vi "Searching connected instruments.vi"(8 "error in (no error)":errorcluster) -> (0 "error out":errorcluster, 2 "Found Instruments":string[][](array[string]))   [LabVIEW 2020, in "Test Framework.lvclass"]
doc: "Finds all connected instruments and gets its IDN.\nFor comport it verifies that a PIC board is connected."
uses:
  Test Framework.lvclass
  <vilib>/Instr/_visa.llb/VISA Find Search Mode.ctl
  <vilib>/Instr/_visa.llb/VISA Configure Serial Port (Instr).vi
panel:
  out "read buffer 2":string
  in  "Cancel":bool
  out "read buffer":string
  out "Searching Instruments":u8(slide) scale=0.0..100.0
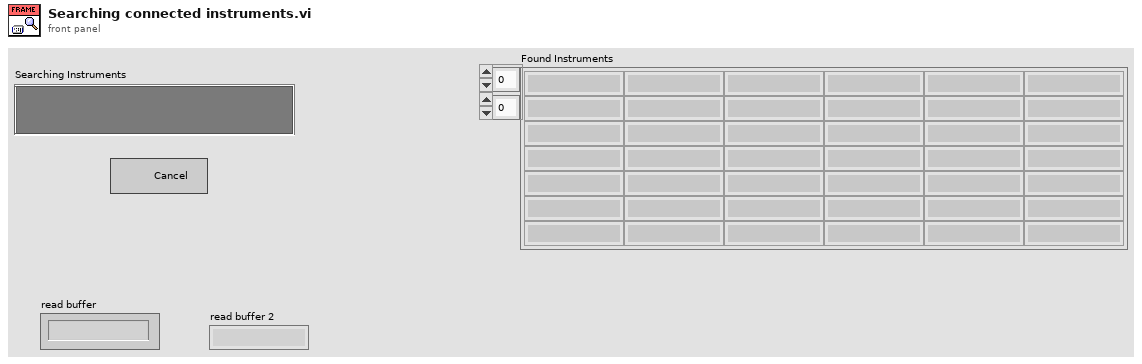
[diagram p1: front panel]
types:
  T1 = typedef "VISA Find Search Mode.ctl" = u32
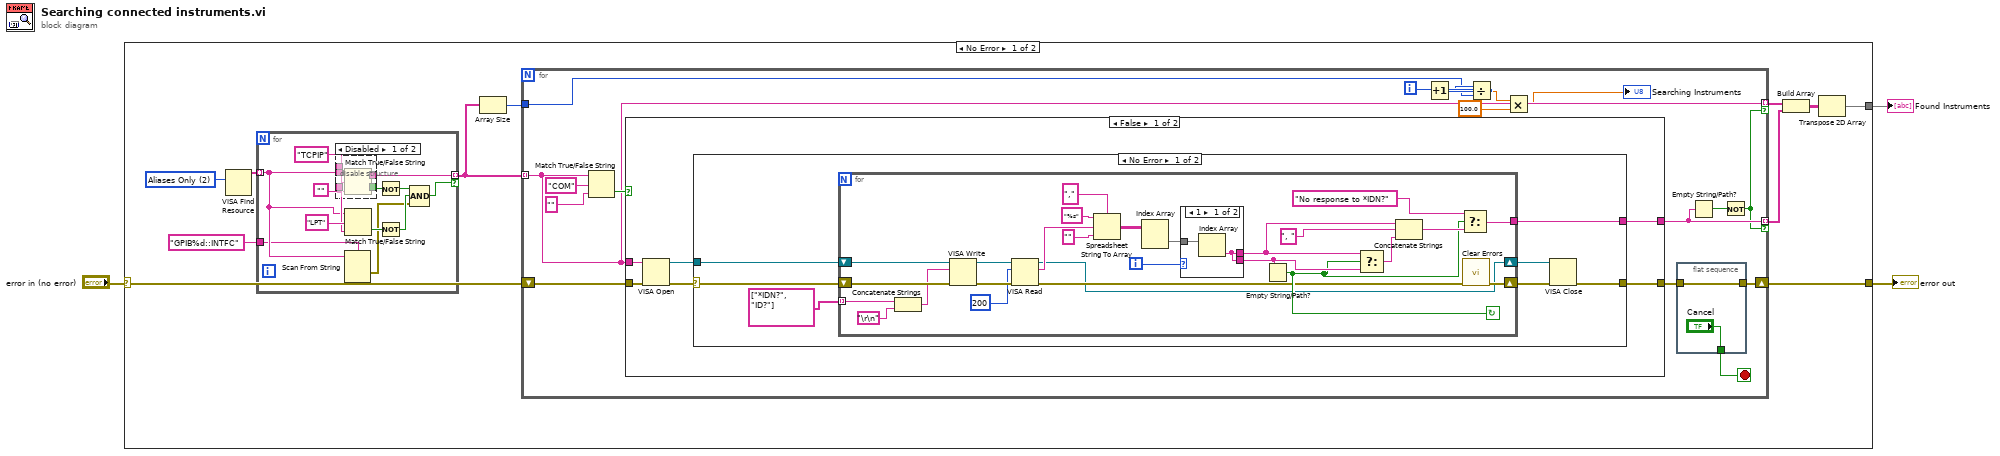
[diagram p0: block diagram]
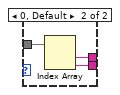
[diagram p2: hidden frame]
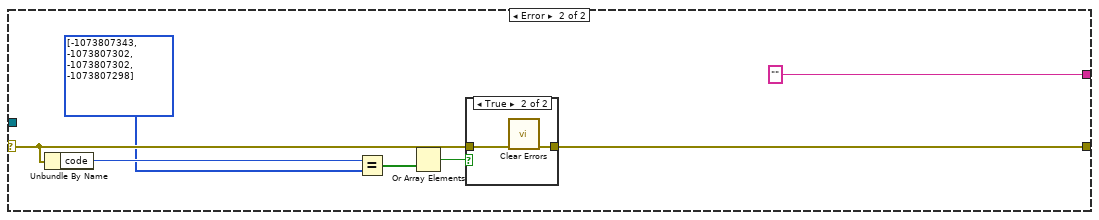
[diagram p3: hidden frame]
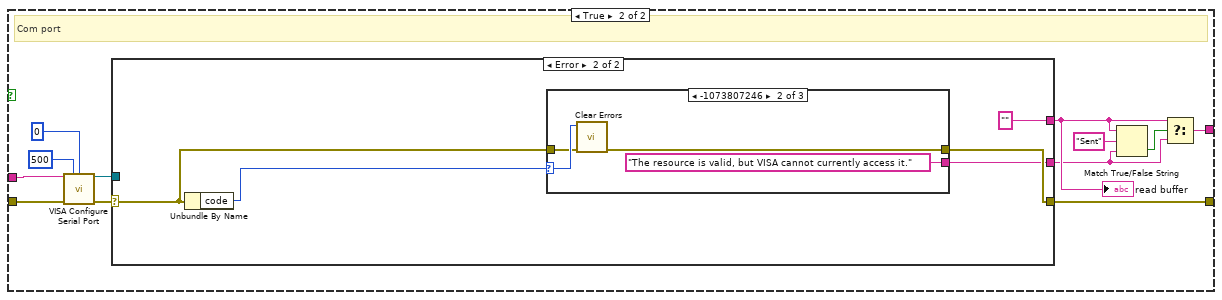
[diagram p5: hidden frame]
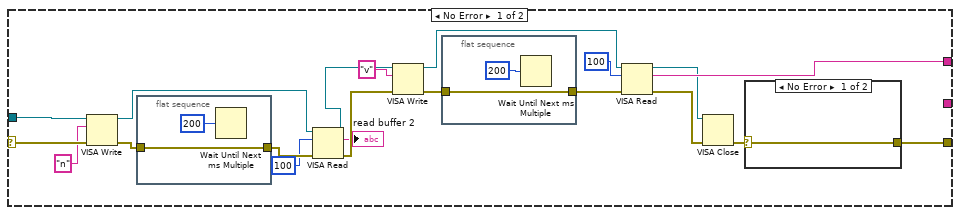
[diagram p6: hidden frame]
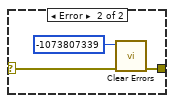
[diagram p7: hidden frame]
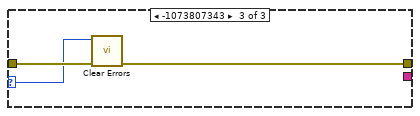
[diagram p9: hidden frame]
diagram:
  n1 = case shown="No Error" "error in (no error)" {
    selector: "error in (no error)" -> [w8 w159]
    tunnel: [w7 w159] -> w2
    tunnel: [w9 _] -> w1
    frame No Error {
      w14 = T1 2 items=["Canonical Names Only"=0, "Aliases Only"=2, "Include Matching Aliases"=3, "Include All Aliases"=4] ("Search Mode")
      n2 = VISA Find Resource(10:w14) -> (3:w13:string[])  [unwired: 2 in, 2 out]
      n3 = for {
        tunnel: w13 -> [w142] mode=indexing
        tunnel: [w152] -> w6 mode=indexing if=w145
        tunnel: "GPIB%d::INTFC" ("true string") -> [w141]
        w144 = ""
        n4 = disable-structure shown="Disabled" {
          disable-tunnel: [w157 w158] -> w152
          disable-tunnel: [w156 _] -> w151
          disable-tunnel: "TCPIP" ("true string") -> [w155 _]
          disable-tunnel: w144 -> [w154 _]
          disable-tunnel: w142 -> [w153 w158]
          frame Disabled {
            n5 = Match True/False String(2:w154, 3:w155, 4:w153) -> (0:w156:bool, 1:w157:string)
          }
          frame Enabled {
          }
        }
        n6 = Scan From String(format string=w141, input string=w142) -> (error out=w143:errorcluster)  [unwired: 4 in, 2 out]
        n7 = Match True/False String(2:w144, 3:"LPT" ("true string"), 4:w142) -> (0:w148:bool)  [unwired: 1 out]
        n8 = Not(x=w151) -> (.not. x?=w147:bool)
        n9 = Not(x=w148) -> (.not. x?=w146:bool)
        n10 = Compound Arithmetic op=AND(w147, w146, w143) -> (w145:bool)
      }
      n11 = Array Size(array=w6) -> (size(s)=w5:i32)
      n12 = for {
        tunnel: w6 -> [w27] mode=indexing
        tunnel: [w26] -> w11 mode=indexing if=w25
        shift-right: [w16] -> w7
        shift-left: w8 -> [w28]
        tunnel: [w27] -> w12 mode=indexing if=w25
        tunnel: w5 -> [w21]
        i -> [w23]
        stop <- w17 stop-if-true
        n13 = Match True/False String(2:"" ("false string"), 3:"COM" ("true string"), 4:w27) -> (0:w29:bool)  [unwired: 1 out]
        n14 = case shown="False" w29 {
          tunnel: w27 -> [w39 w99]
          tunnel: [w37 w91] -> w26
          tunnel: [w35 w94] -> w15
          tunnel: w28 -> [w34 w95]
          frame False {
            n15 = VISA Open(error in (no error)=w34, VISA resource name=w39) -> (VISA resource name=w38:refnum<visa-resource-name>, error out=w36:errorcluster)  [unwired: 3 in]
            n16 = case shown="No Error" w36 {
              selector: w36 -> [w45 w82]
              tunnel: w38 -> [w46 _]
              tunnel: [w44 ""] -> w37
              tunnel: [w41 w81] -> w35
              frame No Error {
                n17 = for {
                  tunnel: [w57] -> w44
                  shift-right: [w59] -> w42
                  shift-left: w45 -> [w62]
                  tunnel: string[] ["*IDN?", "ID?"] -> [w55] mode=indexing
                  shift-right: [w47] -> w40
                  shift-left: w46 -> [w69]
                  i -> [w49]
                  stop <- w50 continue-if-true
                  n18 = Concatenate Strings(w55, "\r\n") -> (w61:string)
                  n19 = VISA Write(VISA resource name=w69, write buffer=w61, error in (no error)=w62) -> (VISA resource name out=w71:refnum<visa-resource-name>, error out=w72:errorcluster)  [unwired: 1 out]
                  n20 = VISA Read(VISA resource name=w71, byte count=u32 200, error in (no error)=w72) -> (VISA resource name out=w47:refnum<visa-resource-name>, read buffer=w51:string, error out=w48:errorcluster)  [unwired: 1 out]
                  n21 = Spreadsheet String To Array(delimiter (Tab)=",", format string="%s", spreadsheet string=w51, array type (2D Dbl)="") -> (array=w66:string[][])
                  n22 = Index Array(array=w66) -> (element=w65:string[])  [unwired: 2 in]
                  n23 = case shown="1" w49 {
                    tunnel: w65 -> [w74 w77]
                    tunnel: [w73 w76] -> w54
                    tunnel: [w73 w75] -> w53
                    frame 1 {
                      n24 = Index Array(array=w74) -> (element=w73:string)  [unwired: 1 in]
                    }
                    frame 0, Default {
                      n25 = Index Array(array=w77) -> (element #1=w76:string, element #2=w75:string)  [unwired: 2 in]
                    }
                  }
                  n26 = Empty String/Path?(string/path=w53) -> (empty?=w50:bool)
                  n27 = Select(t=w54, s=w50, f=w53) -> (s? t:f=w52:string)
                  n28 = Concatenate Strings(w54, ", ", w52) -> (w58:string)
                  n29 = Select(t="No response to *IDN?", s=w50, f=w58) -> (s? t:f=w57:string)
                  n30 = call <vilib>:"Clear Errors.vi"("error in (no error)"=w48) -> ("error out"=w59:errorcluster)  [unwired: 5 in, 1 out]
                }
                n31 = VISA Close(VISA resource name=w40, error in (no error)=w42) -> (error out=w41:errorcluster)
              }
              frame Error {
                n32 = Unbundle By Name(w82) -> ("code"=w83:i32)
                n33 = Equal?(x=w83, y=i32[] [-1073807343, -1073807302, -1073807302, -1073807298]) -> (x = y?=w79:bool[])
                n34 = Or Array Elements(Boolean array=w79) -> (logical OR=w78:bool)
                n35 = case shown="True" w78 {
                  tunnel: w82 -> [w85 w87]
                  tunnel: [w85 w86] -> w81
                  frame False {
                  }
                  frame True {
                    n36 = call <vilib>:"Clear Errors.vi"("error in (no error)"=w87) -> ("error out"=w86:errorcluster)  [unwired: 5 in, 1 out]
                  }
                }
              }
            }
          }
          frame True {
            # "Com port"
            n37 = call-poly "VISA Configure Serial Port"("VISA resource name"=w99, "timeout (10sec)"=u32 500, "termination char\n(0xA = '\\n' = LF)"=u8 0 ("termination char\n(0xA = '\\n' = LF)"), "error in (no error)"=w95) -> ("VISA resource name out"=w97:refnum<visa-resource-name>, "error out"=w96:errorcluster)  [unwired: 10 in]
            n38 = case shown="Error" w96 {
              selector: w96 -> [w109 w132]
              tunnel: w97 -> [w108 _]
              tunnel: [w117 "" ("message")] -> w89
              tunnel: [w110 w131] -> w94
              tunnel: [_ w129] -> w88
              frame No Error {
                n39 = VISA Write(VISA resource name=w108, write buffer="n", error in (no error)=w109) -> (VISA resource name out=w105:refnum<visa-resource-name>, error out=w107:errorcluster)  [unwired: 1 out]
                n40 = flat-sequence {
                  tunnel: [w120] -> w106
                  tunnel: w107 -> [w120]
                  frame #0 {
                    n41 = Wait Until Next ms Multiple(millisecond multiple=u32 200) -> ()  [unwired: 1 out]
                  }
                }
                n42 = VISA Read(VISA resource name=w105, byte count=u32 100, error in (no error)=w106) -> (VISA resource name out=w103:refnum<visa-resource-name>, read buffer=→"read buffer 2":string, error out=w102:errorcluster)  [unwired: 1 out]
                n43 = VISA Write(VISA resource name=w103, write buffer="v", error in (no error)=w102) -> (VISA resource name out=w114:refnum<visa-resource-name>, error out=w115:errorcluster)  [unwired: 1 out]
                n44 = flat-sequence {
                  tunnel: [w126] -> w116
                  tunnel: w115 -> [w126]
                  frame #0 {
                    n45 = Wait Until Next ms Multiple(millisecond multiple=u32 200) -> ()  [unwired: 1 out]
                  }
                }
                n46 = VISA Read(VISA resource name=w114, byte count=u32 100, error in (no error)=w116) -> (VISA resource name out=w112:refnum<visa-resource-name>, read buffer=w117:string, error out=w113:errorcluster)  [unwired: 1 out]
                n47 = VISA Close(VISA resource name=w112, error in (no error)=w113) -> (error out=w111:errorcluster)
                n48 = case shown="No Error" w111 {
                  selector: w111 -> [w122 w124]
                  tunnel: [w122 w125] -> w110
                  frame No Error {
                  }
                  frame Error {
                    n49 = call <vilib>:"Clear Errors.vi"("error in (no error)"=w124, "specific error code to clear (0: all)"=-1073807339) -> ("error out"=w125:errorcluster)  [unwired: 4 in, 1 out]
                  }
                }
              }
              frame Error {
                n50 = Unbundle By Name(w132) -> ("code"=w130:i32)
                n51 = case shown="-1073807246" w130 {
                  selector: w130 -> [_ w137 w138]
                  tunnel: w132 -> [w133 w135 w140]
                  tunnel: [w133 w136 w139] -> w131
                  tunnel: [_ "The resource is valid, but VISA cannot currently access it." ("false string") _] -> w129
                  frame 0, Default {
                  }
                  frame -1073807246 {
                    n52 = call <vilib>:"Clear Errors.vi"("error in (no error)"=w135, "specific error code to clear (0: all)"=w137) -> ("error out"=w136:errorcluster)  [unwired: 4 in, 1 out]
                  }
                  frame -1073807343 {
                    n53 = call <vilib>:"Clear Errors.vi"("error in (no error)"=w140, "specific error code to clear (0: all)"=w138) -> ("error out"=w139:errorcluster)  [unwired: 4 in, 1 out]
                  }
                }
              }
            }
            "read buffer" <- w89
            n54 = Match True/False String(2:w88, 3:"Sent" ("true string"), 4:w89) -> (0:w92:bool)  [unwired: 1 out]
            n55 = Select(t=w89, s=w92, f=w88) -> (s? t:f=w91:string)
          }
        }
        n56 = Increment(x=w23) -> (x+1=w22:i32)
        n57 = Divide(x=w22, y=w21) -> (x/y=w20:dbl)
        n58 = Multiply(x=w20, y=100.0) -> (x*y=→"Searching Instruments":dbl)
        n59 = flat-sequence {
          tunnel: ["Cancel"] -> w17
          tunnel: w15 -> [w32]
          tunnel: [w32] -> w16
          frame #0 {
          }
        }
        n60 = Empty String/Path?(string/path=w26) -> (empty?=w24:bool)
        n61 = Not(x=w24) -> (.not. x?=w25:bool)
      }
      n62 = Build Array(w12, w11) -> (w10:string[][])
      n63 = Transpose 2D Array(2D array=w10) -> (transposed array=w9:string[][])
    }
    frame Error {
    }
  }
  "error out" <- w2
  "Found Instruments" <- w1
